vi "script user process vi.vi"(8 "error in":errorcluster, 10 "runtime class path in":path, 11 "Application in":refnum<vi>) -> (0 "error out":errorcluster)   [LabVIEW 2013]
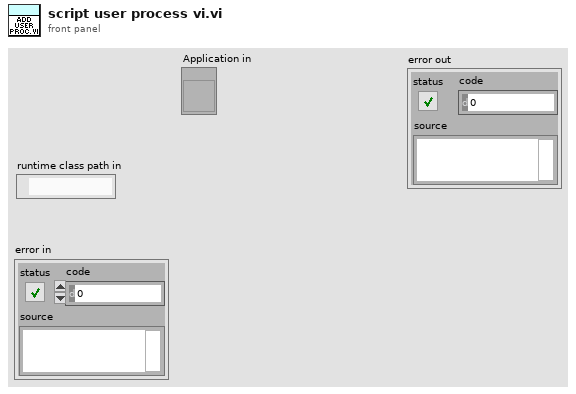
[diagram p1: front panel]
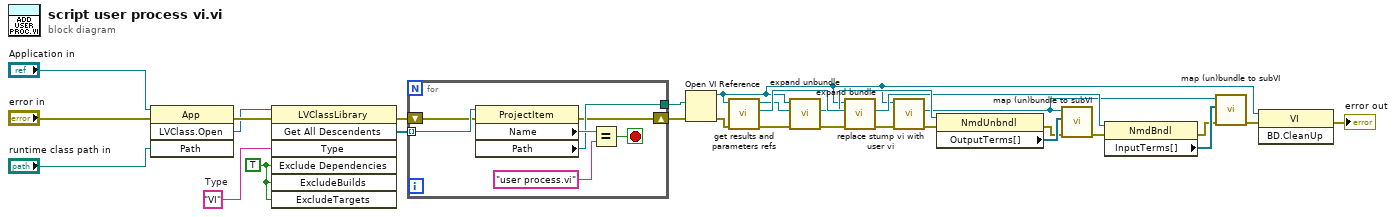
[diagram p0: block diagram]
diagram:
  w28 = TRUE
  w27 = "VI"  # Type
  n1 = invoke class="App" method="LVClass.Open"(reference="Application in", error in="error in", "Path"="runtime class path in") -> (error out=w29:errorcluster, "LVClass.Open"=w26:refnum<vi>)  [unwired: 1 in, 2 out]
  n2 = invoke class="LVClassLibrary" method="Get All Descendents"(reference=w26, error in=w29, "Type"=w27, "Exclude Dependencies"=w28, "ExcludeBuilds"=w28, "ExcludeTargets"=w28) -> (error out=w20:errorcluster, "All Descendents"=w22:refnum<vi>[])  [unwired: 1 in, 5 out]
  n3 = for {
    tunnel: w22 -> [w33] mode=indexing
    tunnel: [w32] -> w21
    shift-right: [w31] -> w18
    shift-left: w20 -> [w30]
    stop <- w34 stop-if-true
    n4 = property class="ProjectItem"(reference=w33, error in=w30) -> (error out=w31:errorcluster, "Name"=w36:string, "Path"=w32:path)  [unwired: 1 out]
    n5 = Equal?(x=w36, y="user process.vi") -> (x = y?=w34:bool)
  }
  n6 = Open VI Reference(vi path=w21, error in (no error)=w18) -> (vi reference=w3:refnum<vi>, error out=w19:errorcluster)  [unwired: 4 in]
  n7 = call "get results and parameters refs.vi"("error in"=w19, "VI in"=w3) -> ("error out"=w15:errorcluster, "Results from processing ref out"=w17:refnum<vi>, "Parameters to process ref out"=w16:refnum<vi>)  [unwired: 7 in]
  n8 = call "expand unbundle.vi"("error in"=w15, "Parameters to process ref in"=w16, "VI Refnum"=w3) -> ("error out"=w14:errorcluster, "unbundle ref out"=w12:refnum<vi>)  [unwired: 7 in]
  n9 = call "expand bundle.vi"("error in (no error)"=w14, "Results from processing ref in"=w17, "VI Refnum"=w3) -> ("error out"=w13:errorcluster, "Bundle ref out"=w8:refnum<vi>)  [unwired: 7 in]
  n10 = call "replace stump vi with user vi.vi"("error in (no error)"=w13, "VI in"=w3) -> ("error out"=w10:errorcluster, "subvi reference out"=w6:refnum<vi>)  [unwired: 8 in]
  n11 = property class="NmdUnbndl"(reference=w12, error in=w10) -> (error out=w9:errorcluster, "OutputTerms[]"=w11:refnum<vi>[])  [unwired: 1 out]
  n12 = call "map (un)bundle to subVI.vi"("error in (no error)"=w9, "Terms[]"=w11, "SubVI in"=w6) -> ("error out"=w5:errorcluster)  [unwired: 8 in]
  n13 = property class="NmdBndl"(reference=w8, error in=w5) -> (error out=w4:errorcluster, "InputTerms[]"=w7:refnum<vi>[])  [unwired: 1 out]
  n14 = call "map (un)bundle to subVI.vi"("error in (no error)"=w4, "Terms[]"=w7, "SubVI in"=w6) -> ("error out"=w2:errorcluster)  [unwired: 8 in]
  n15 = invoke class="VI" method="BD.CleanUp"(reference=w3, error in=w2) -> (error out=→"error out":errorcluster)  [unwired: 1 in, 2 out]
